vi "HFRR ADV v06 new software.vi"() -> ()   [LabVIEW 2025] (continued)
            frame 13 {
              n1278 = local write "CH-HEATER"(w1592) -> ()
            }
            frame 14 {
              n1279 = local write "CH-HUMIDITY WET"(w1593) -> ()
            }
            frame 15 {
              n1280 = local write "CH-HUMIDITY DRY"(w1594) -> ()
            }
            frame 16 {
            }
            frame 17 {
              n1281 = local write "AIR TEMP INTERCEPT:"(w1595) -> ()
            }
            frame 18 {
              n1282 = local write "TEMP INTERCEPT:"(w1596) -> ()
            }
            frame 19 {
              n1283 = local write "S.NO"(w1597) -> ()
            }
            frame 20 {
              n1284 = local write "Com Port 3"(w1598) -> ()
            }
            frame 21 {
            }
            frame 22 {
              n1285 = local write "C3 :"(w1599) -> ()
            }
            frame 23, Default {
            }
          }
        }
      }
    }
    n1286 = Select(t=u32 2500 ("milliseconds to wait"), s=w1553, f=u32 500 ("milliseconds to wait")) -> (s? t:f=w1551:u32)
    n1287 = Multiply(x=w1556, y=w1551) -> (x*y=w1558:dbl)
    n1288 = property on="Time slide" class="Slide (strict)"("Visible"=w1547) -> ()  [unwired: 2 in, 2 out]
    n1289 = call "Elapsed Time2"("Time Target (s)"=w1558, "Auto Reset"=TRUE) -> ("Time has Elapsed"=w1548:bool)  [unwired: 10 in, 7 out]
    n1290 = case shown="True" w1548 {
      frame False {
      }
      frame True {
        n1291 = stacked-sequence {
          frame #0 {
            # "DATA PROCESSING"
            # "115 mV/N"
            n1292 = local read "Sample Temperature"() -> (w1600:dbl)
            "TEMP 2" <- w1600
            "TEMP 3" <- w1600
            n1293 = local read "RH Numeric:"() -> (w1607:dbl)
            n1294 = local read "HUMIDITY:"() -> (w1608:dbl)
            n1295 = local read "FRICVALZ"() -> (w1619:dbl)
            n1296 = local read "Friction"() -> (w1603:dbl)
            n1297 = local write "TEMP"(w1600) -> ()
            n1298 = Multiply(x=w1607, y=w1608) -> (x*y=→"Humidity ( %RH )" →"Hum" →"Hum 2":dbl)
            n1299 = Subtract(x=w1603, y=w1619) -> (x-y=w1614:dbl)
            "FF 2" <- w1614
            "FF 4" <- w1614
            n1300 = local read "Ambient Temperature"() -> (→"AIR TEMP":dbl)
            n1301 = local read "TEMP"() -> (w1618:dbl)
            n1302 = local write "FF 3"(w1614) -> ()
            n1303 = Compound Arithmetic op=OR("FRICVALZ 4", "FRICVALZ 3", "FRICVALZ 2") -> (w1610:bool)
            n1304 = case shown="True" w1610 {
              tunnel: w1603 -> [_ w1625]
              frame False {
              }
              frame True {
                w1624 = FALSE ("FRICVALZ")
                n1305 = local write "FRICVALZ 3"(w1624) -> ()
                n1306 = local write "FRICVALZ 2"(w1624) -> ()
                n1307 = local write "FRICVALZ 4"(w1624) -> ()
                "FRICVALZ" <- w1625
              }
            }
            n1308 = Not A Number/Path/Refnum?(number/path/refnum=w1618) -> (NaN/Path/Refnum?=w1617:bool)
            n1309 = Not A Number/Path/Refnum?(number/path/refnum=w1614) -> (NaN/Path/Refnum?=w1616:bool)
            n1310 = Divide(x=w1614, y=1.96) -> (x/y=w1611:dbl)
            n1311 = Compound Arithmetic op=OR(w1617, w1616) -> (w1615:bool)
            n1312 = Not A Number/Path/Refnum?(number/path/refnum=w1611) -> (NaN/Path/Refnum?=w1612:bool)
            n1313 = case shown="True" w1615 {
              frame False {
              }
              frame True {
                n1314 = local write "TEMP"(0.0 ("TEMP")) -> ()
                n1315 = local write "FF 2"(0.0 ("FF 2")) -> ()
                n1316 = local write "reinit"(TRUE ("reinit")) -> ()
              }
            }
            n1317 = Select(t=0.0, s=w1612, f=w1611) -> (s? t:f=w1602:dbl)
            "COF 2" <- w1602
            n1318 = local write "COF 3"(w1602) -> ()
          }
        }
      }
    }
    n1319 = Wait (ms)(milliseconds to wait=u32 50) -> ()  [unwired: 1 out]
    n1320 = local read "Quit"() -> (w1540:bool)
    "Rate" <- 2500.0 ("No of Samples")
  }
  n1321 = while {
    tunnel: w57 -> [_]
    tunnel: [w1652] -> _
    tunnel: [w1628] -> w56
    i -> [w1652]
    stop <- w1628 stop-if-true
    # "C:\\LAB-IQ-NXT\\Scar View.exe"
    n1322 = local read "OK Button 16"() -> (w1641:bool)
    n1323 = local read "Main Tab"() -> (w1634:T2)
    n1324 = local read "service 3"() -> (w1635:bool)
    n1325 = local read "OPEN 6"() -> (w1637:bool)
    n1326 = local read "EDIT 2"() -> (w1639:bool)
    n1327 = flat-sequence {
      frame #0 {
        n1328 = local read "SAVE 2"() -> (w2254:bool)
        n1329 = stacked-sequence {
          frame #0 {
            n1330 = local read "EDIT"() -> (w2308:bool)
            n1331 = case shown="True" w2308 {
              tunnel: [u8 2 ("Disabled") u8 0 ("Disabled")] -> _
              frame False {
                w2310 = FALSE
                n1332 = local write "Password"("") -> ()
                n1333 = property on="SrvM CP" class="Bool (strict)"("Visible"=w2310) -> ()  [unwired: 2 in, 2 out]
                n1334 = property on="message" class="Str"("Visible"=w2310) -> ()  [unwired: 2 in, 2 out]
                n1335 = local write "x = y?"(w2310) -> ()
                n1336 = property on="Password" class="Str"("Visible"=w2310) -> ()  [unwired: 2 in, 2 out]
                n1337 = property on="ENTER THE NEW PASSWORD" class="Str"("Visible"=w2310) -> ()  [unwired: 2 in, 2 out]
                n1338 = property on="ENTER CURRENT PASSWORD" class="Str"("Visible"=w2310) -> ()  [unwired: 2 in, 2 out]
                n1339 = local write "SrvM CP"(w2310) -> ()
              }
              frame True {
                w2313 = TRUE
                n1340 = property on="SrvM CP" class="Bool (strict)"("Visible"=w2313) -> ()  [unwired: 2 in, 2 out]
                n1341 = property on="Password" class="Str"("Visible"=w2313) -> ()  [unwired: 2 in, 2 out]
              }
            }
            "dipl pwd" <- "@143$\n" ("dipl pwd")
          }
          frame #1 {
            # "Gain password"
            n1342 = String To Byte Array(string="ENTER CURRENT PASSWORD") -> (unsigned byte array=w2318:u8[])
            n1343 = Search 1D Array(1D array=w2318, element=u8 10) -> (index of element=w2321:i32)  [unwired: 1 in]
            n1344 = Index Array(array=w2318, index=w2321) -> (element=w2317:u8)
            n1345 = Equal?(x=w2317, y=10) -> (x = y?=w2315:bool)
            n1346 = case shown="True" w2315 {
              frame False {
                n1347 = property on="ENTER THE NEW PASSWORD" class="Str"("Visible"=FALSE) -> ()  [unwired: 2 in, 2 out]
              }
              frame True {
                # "password"
                # "change password logic"
                n1348 = local read "ENTER CURRENT PASSWORD"() -> (w2334:string)
                n1349 = local read "dipl pwd"() -> (w2328:string)
                n1350 = String To Byte Array(string=w2334) -> (unsigned byte array=w2336:u8[])
                n1351 = String To Byte Array(string=w2328) -> (unsigned byte array=w2329:u8[])
                n1352 = Array Size(array=w2336) -> (size(s)=w2333:i32)
                n1353 = Array Size(array=w2329) -> (size(s)=w2331:i32)
                n1354 = for {
                  N: w2333 -> [_]
                  tunnel: w2336 -> [w2360]
                  tunnel: [w2358] -> w2337 mode=indexing
                  tunnel: w2333 -> [w2352]
                  i -> [w2353]
                  n1355 = Decrement(x=w2352) -> (x-1=w2350:i32)
                  n1356 = Equal?(x=w2353, y=w2350) -> (x = y?=w2351:bool)
                  n1357 = Index Array(array=w2360, index=w2353) -> (element=w2354:u8)
                  n1358 = Number To Decimal String(number=w2354) -> (decimal integer string=w2359:string)  [unwired: 1 in]
                  n1359 = Select(t="", s=w2351, f="\r") -> (s? t:f=w2356:string)
                  n1360 = Concatenate Strings(w2359, w2356) -> (w2358:string)
                }
                n1361 = for {
                  N: w2331 -> [_]
                  tunnel: w2329 -> [w2348]
                  tunnel: [w2346] -> w2330 mode=indexing
                  tunnel: w2331 -> [w2343]
                  i -> [w2344]
                  n1362 = Decrement(x=w2343) -> (x-1=w2342:i32)
                  n1363 = Equal?(x=w2344, y=w2342) -> (x = y?=w2341:bool)
                  n1364 = Index Array(array=w2348, index=w2344) -> (element=w2347:u8)
                  n1365 = Number To Decimal String(number=w2347) -> (decimal integer string=w2345:string)  [unwired: 1 in]
                  n1366 = Select(t="", s=w2341, f="\r") -> (s? t:f=w2338:string)
                  n1367 = Concatenate Strings(w2345, w2338) -> (w2346:string)
                }
                n1368 = local read "string"() -> (w2335:string)
                n1369 = Concatenate Strings(w2330) -> (w2324:string)
                n1370 = Concatenate Strings(w2335) -> (w2332:string)
                n1371 = Concatenate Strings(w2337) -> (w2325:string)
                n1372 = Equal?(x=w2325, y=w2332) -> (x = y?=w2327:bool)
                n1373 = Equal?(x=w2325, y=w2324) -> (x = y?=w2323:bool)
                n1374 = Or(x=w2327, y=w2323) -> (x .or. y?=w2326:bool)
                n1375 = case shown="True" w2326 {
                  frame False {
                  }
                  frame True {
                    n1376 = property on="ENTER THE NEW PASSWORD" class="Str"("Visible"=TRUE) -> ()  [unwired: 2 in, 2 out]
                  }
                }
              }
            }
          }
          frame #2 {
            n1377 = String To Byte Array(string="ENTER THE NEW PASSWORD") -> (unsigned byte array=w2363:u8[])
            n1378 = Search 1D Array(1D array=w2363, element=u8 10) -> (index of element=w2367:i32)  [unwired: 1 in]
            n1379 = Index Array(array=w2363, index=w2367) -> (element=w2365:u8)
            n1380 = Equal?(x=w2365, y=10) -> (x = y?=w2362:bool)
            n1381 = case shown="False" w2362 {
              frame False {
              }
              frame True {
                n1382 = local write "EDIT"(FALSE) -> ()
                n1383 = local write "SrvM CP"(FALSE) -> ()
                n1384 = local read "ENTER THE NEW PASSWORD"() -> (w2370:string)
                n1385 = String To Byte Array(string=w2370) -> (unsigned byte array=w2375:u8[])
                n1386 = Array Size(array=w2375) -> (size(s)=w2372:i32)
                n1387 = for {
                  N: w2372 -> [_]
                  tunnel: w2375 -> [w2388]
                  tunnel: [w2385] -> w2377 mode=indexing
                  tunnel: w2372 -> [w2380]
                  i -> [w2378]
                  n1388 = Decrement(x=w2380) -> (x-1=w2381:i32)
                  n1389 = Equal?(x=w2378, y=w2381) -> (x = y?=w2382:bool)
                  n1390 = Index Array(array=w2388, index=w2378) -> (element=w2387:u8)
                  n1391 = Number To Decimal String(number=w2387) -> (decimal integer string=w2386:string)  [unwired: 1 in]
                  n1392 = Select(t="", s=w2382, f="\r") -> (s? t:f=w2379:string)
                  n1393 = Concatenate Strings(w2386, w2379) -> (w2385:string)
                }
                n1394 = local read "file path"() -> (w2369:path)
                n1395 = Concatenate Strings(w2377) -> (w2371:string)
                n1396 = Delete(path (use dialog)=w2369) -> (deleted path=w2373:path)  [unwired: 4 in, 2 out]
                n1397 = call <vilib>:"Write Characters To File.vi"("append to file? (new file:F)"=FALSE, "character string"=w2371, "file path (dialog if empty)"=w2373) -> ()  [unwired: 2 in, 1 out]
              }
            }
          }
          frame #3 {
            n1398 = case shown="True" "SrvM CP" {
              frame False {
                w2391 = ""
                n1399 = local write "ENTER CURRENT PASSWORD"(w2391) -> ()
                n1400 = local write "ENTER THE NEW PASSWORD"(w2391) -> ()
                n1401 = property on="ENTER CURRENT PASSWORD" class="Str"("Visible"=FALSE) -> ()  [unwired: 2 in, 2 out]
              }
              frame True {
                n1402 = property on="ENTER THE NEW PASSWORD" class="Str"() -> ("Visible"=w2392:bool)  [unwired: 2 in, 2 out]
                n1403 = Not(x=w2392) -> (.not. x?=w2393:bool)
                n1404 = property on="ENTER CURRENT PASSWORD" class="Str"("Visible"=w2393) -> ()  [unwired: 2 in, 2 out]
              }
            }
          }
          frame #4 {
            n1405 = String To Byte Array(string="Password") -> (unsigned byte array=w2400:u8[])
            n1406 = Search 1D Array(1D array=w2400, element=u8 10) -> (index of element=w2398:i32)  [unwired: 1 in]
            n1407 = Index Array(array=w2400, index=w2398) -> (element=w2399:u8)
            n1408 = Equal?(x=w2399, y=10) -> (x = y?=w2395:bool)
            n1409 = case shown="True" w2395 {
              frame False {
              }
              frame True {
                # "password"
                # "password"
                n1410 = local read "Password"() -> (w2413:string)
                n1411 = String To Byte Array(string=w2413) -> (unsigned byte array=w2416:u8[])
                n1412 = String To Byte Array(string="@143$\n") -> (unsigned byte array=w2402:u8[])
                n1413 = Array Size(array=w2416) -> (size(s)=w2411:i32)
                n1414 = Array Size(array=w2402) -> (size(s)=w2407:i32)
                n1415 = for {
                  N: w2411 -> [_]
                  tunnel: w2416 -> [w2450]
                  tunnel: [w2448] -> w2417 mode=indexing
                  tunnel: w2411 -> [w2445]
                  i -> [w2446]
                  n1416 = Decrement(x=w2445) -> (x-1=w2444:i32)
                  n1417 = Index Array(array=w2450, index=w2446) -> (element=w2449:u8)
                  n1418 = Equal?(x=w2446, y=w2444) -> (x = y?=w2443:bool)
                  n1419 = Number To Decimal String(number=w2449) -> (decimal integer string=w2447:string)  [unwired: 1 in]
                  n1420 = Select(t="", s=w2443, f="\r") -> (s? t:f=w2440:string)
                  n1421 = Concatenate Strings(w2447, w2440) -> (w2448:string)
                }
                n1422 = for {
                  N: w2407 -> [_]
                  tunnel: w2402 -> [w2461]
                  tunnel: [w2459] -> w2405 mode=indexing
                  tunnel: w2407 -> [w2456]
                  i -> [w2457]
                  n1423 = Decrement(x=w2456) -> (x-1=w2455:i32)
                  n1424 = Index Array(array=w2461, index=w2457) -> (element=w2460:u8)
                  n1425 = Equal?(x=w2457, y=w2455) -> (x = y?=w2454:bool)
                  n1426 = Number To Decimal String(number=w2460) -> (decimal integer string=w2458:string)  [unwired: 1 in]
                  n1427 = Select(t="", s=w2454, f="\r") -> (s? t:f=w2451:string)
                  n1428 = Concatenate Strings(w2458, w2451) -> (w2459:string)
                }
                n1429 = local read "file path"() -> (w2401:path)
                n1430 = call <vilib>:"Read Characters From File.vi"("file path (dialog if empty)"=w2401) -> ("character string"=w2415:string)  [unwired: 5 in, 3 out]
                "string" <- w2415
                n1431 = flat-sequence {
                  tunnel: [w2418] -> w2412
                  frame #0 {
                    w2418 = ""
                    n1432 = local write "Password"(w2418) -> ()
                  }
                }
                n1433 = Concatenate Strings(w2405) -> (w2406:string)
                n1434 = Concatenate Strings(w2415) -> (w2414:string)
                n1435 = Concatenate Strings(w2417) -> (w2409:string)
                n1436 = Equal?(x=w2409, y=w2414) -> (x = y?=w2404:bool)
                n1437 = Equal?(x=w2409, y=w2406) -> (x = y?=w2410:bool)
                n1438 = Or(x=w2404, y=w2410) -> (x .or. y?=w2403:bool)
                "x = y?" <- w2403
                n1439 = case shown="True" w2403 {
                  selector: w2403 -> [w2420 _]
                  tunnel: w2412 -> [_ _]
                  frame False {
                    n1440 = And(x=w2420, y=TRUE ("Visible")) -> (x .and. y?=w2421:bool)
                    n1441 = property on="message" class="Str"("Visible"=w2421) -> ()  [unwired: 2 in, 2 out]
                  }
                  frame True {
                    n1442 = control-ref of="This VI"() -> (w2432:refnum<vi>)
                    n1443 = property class="VI"(reference=w2432) -> (reference out=w2423:refnum<vi>, error out=w2427:errorcluster, "Panel"=w2431:refnum<vi>)  [unwired: 1 in]
                    n1444 = property on="message" class="Str"("Visible"=FALSE) -> ()  [unwired: 2 in, 2 out]
                    n1445 = property class="Pnl"(reference=w2431, error in=w2427) -> (reference out=w2425:refnum<vi>, error out=w2428:errorcluster, "Panes[]"=w2430:refnum<vi>[])
                    n1446 = for {
                      tunnel: w2430 -> [w2439] mode=indexing
                      tunnel: T16."Always On" ("Horizontal Scrollbar Visibility") -> [w2438]
                      tunnel: w2428 -> [w2435]
                      tunnel: [w2434] -> w2426
                      n1447 = property class="Pane"(reference=w2439, error in=w2435, "HorizScrollbarVisibility"=w2438) -> (reference out=w2436:refnum<vi>, error out=w2437:errorcluster)
                      n1448 = Close Reference(reference=w2436, error in (no error)=w2437) -> (error out=w2434:errorcluster)
                    }
                    n1449 = Close Reference(reference=w2425, error in (no error)=w2426) -> (error out=w2424:errorcluster)
                    n1450 = Close Reference(reference=w2423, error in (no error)=w2424) -> (error out=→"error out 6":errorcluster)
                  }
                }
              }
            }
          }
        }
        n1451 = local read "x = y?"() -> (w2260:bool)
        n1452 = local read "HUMIDITY: 2"() -> (w2262:dbl)
        n1453 = local read "HUMIDITY:"() -> (w2261:dbl)
        n1454 = property on="Port 2 Error" class="Clust (strict)"("Visible"="EDIT") -> ()  [unwired: 2 in, 2 out]
        n1455 = property on="Port 1 Error" class="Clust (strict)"("Visible"="EDIT") -> ()  [unwired: 2 in, 2 out]
        n1456 = case shown="True" "SrvM CP 2" {
          frame False {
          }
          frame True {
            n1457 = local write "SrvM CP 2"(FALSE ("SrvM CP 2")) -> ()
            n1458 = local read "HUMIDITY: 2"() -> (w2301:dbl)
            n1459 = local read "TEMP INTERCEPT: 2"() -> (w2300:dbl)
            n1460 = local read "DISPLACEMENT : 4"() -> (w2304:dbl)
            n1461 = local read "TEMPERATURE : 2"() -> (w2303:dbl)
            n1462 = local read "STROKE GAIN : 2"() -> (w2305:dbl)
            n1463 = local read "FRIC. FORCE : 2"() -> (w2306:dbl)
            n1464 = local read "AIR TEMP INTERCEPT: 2"() -> (w2299:dbl)
            n1465 = local read "AIR TEMPERATURE : 2"() -> (w2302:dbl)
            n1466 = local write "HUMIDITY:"(w2301) -> ()
            n1467 = local write "AIR TEMP INTERCEPT:"(w2300) -> ()
            n1468 = local write "TEMPERATURE :"(w2303) -> ()
            n1469 = local write "FRIC. FORCE :"(w2306) -> ()
            n1470 = local write "STROKE GAIN :"(w2305) -> ()
            n1471 = local write "DISPLACEMENT :"(w2304) -> ()
            n1472 = local write "AIR TEMPERATURE :"(w2302) -> ()
            n1473 = local write "TEMP INTERCEPT:"(w2299) -> ()
          }
        }
        n1474 = Or(x="SAVE", y=w2254) -> (x .or. y?=w2255:bool)
        n1475 = And(x="EDIT", y=w2260) -> (x .and. y?=w2258:bool)
        n1476 = local read "DISPLACEMENT : 4"() -> (w2271:dbl)
        n1477 = local read "TEMPERATURE : 2"() -> (w2269:dbl)
        n1478 = local read "STROKE GAIN : 2"() -> (w2275:dbl)
        n1479 = local read "DISPLACEMENT :"() -> (w2270:dbl)
        n1480 = local read "FRIC. FORCE : 2"() -> (w2278:dbl)
        n1481 = local read "TEMPERATURE :"() -> (w2267:dbl)
        n1482 = local read "STROKE GAIN :"() -> (w2274:dbl)
        n1483 = local read "FRIC. FORCE :"() -> (w2277:dbl)
        n1484 = case shown="True" w2258 {
          tunnel: [u8 2 ("Disabled") u8 0 ("Disabled")] -> w2257
          tunnel: [w2622 TRUE ("Visible")] -> w2256
          frame False {
            w2622 = FALSE ("Visible")
            n1485 = local write "EDIT 2"(w2622) -> ()
          }
          frame True {
          }
        }
        n1486 = case shown="True" w2255 {
          frame False {
          }
          frame True {
            n1487 = stacked-sequence {
              seq-local: [w2470 _ _] -> [_ w2617 _]
              frame #0 {
                (unwired) i16 5 ("precision (6)")
                # "[CH1]    - FF\n[CH2]   - TEMPERATURE\n[CH3]    - Humidity\n[CH4]    - AIR TEMP\n[CH5]\\- Visa Uno\n[CH6] \\- Visa Due\n[CH7]  \\- file path\n[CH8]   - Displacement Gain\n[CHA]   - Stroke Gain\n[CHB]   - Stroke PID Gain\n[CHC]   -Language Selection\n[CHD]   -Power +\n[CHE]   -Power_\n[CHF]   -Heater\n[CHG]   -Humidity Wet\n[CHH]   -Humidity Dry\n[CHI]   -Integral Time"
                n1488 = local read "Language Selection"() -> (w2518:enum16{"English", "Russian"})
                n1489 = local read "CH-HUMIDITY WET"() -> (w2476:u16)
                n1490 = local read "CH-HUMIDITY DRY"() -> (w2473:u16)
                n1491 = local read "STROKE GAIN :"() -> (w2462:dbl)
                n1492 = local read "CH-POWER +"() -> (w2485:u16)
                n1493 = local read "CH-POWER -"() -> (w2482:u16)
                n1494 = local read "CH-HEATER"() -> (w2479:u16)
                n1495 = local read "AIR TEMPERATURE :"() -> (w2465:dbl)
                n1496 = local read "DISPLACEMENT :"() -> (w2463:dbl)
                n1497 = local read "TEMPERATURE :"() -> (w2466:dbl)
                n1498 = local read "FRIC. FORCE :"() -> (w2467:dbl)
                n1499 = local read "HUMIDITY:"() -> (w2464:dbl)
                n1500 = Path To String(path="File Path") -> (string=w2534:string)
                n1501 = Number To Fractional String(number=w2462, width (-)=i16 10 ("precision (6)"), precision (6)=i16 5) -> (F-format string=w2525:string)  [unwired: 1 in]
                n1502 = Number To Fractional String(number=w2518, width (-)=i16 10 ("precision (6)"), precision (6)=i16 5) -> (F-format string=w2514:string)  [unwired: 1 in]
                n1503 = Number To Fractional String(number=w2485, width (-)=i16 10 ("precision (6)"), precision (6)=i16 5) -> (F-format string=w2508:string)  [unwired: 1 in]
                n1504 = Number To Fractional String(number=w2482, width (-)=i16 10 ("precision (6)"), precision (6)=i16 5) -> (F-format string=w2505:string)  [unwired: 1 in]
                n1505 = Number To Fractional String(number=w2479, width (-)=i16 10 ("precision (6)"), precision (6)=i16 5) -> (F-format string=w2500:string)  [unwired: 1 in]
                n1506 = Number To Fractional String(number=w2476, width (-)=i16 10 ("precision (6)"), precision (6)=i16 5) -> (F-format string=w2497:string)  [unwired: 1 in]
                n1507 = Number To Fractional String(number=w2473, width (-)=i16 10 ("precision (6)"), precision (6)=i16 5) -> (F-format string=w2492:string)  [unwired: 1 in]
                n1508 = local read "Com Port 1"() -> (w2469:refnum<visa-resource-name>)
                n1509 = local read "Com Port 2"() -> (w2468:refnum<visa-resource-name>)
                n1510 = Concatenate Strings(w2534, "\\" ("string")) -> (w2533:string)
                n1511 = Number To Fractional String(number=w2467, width (-)=i16 10 ("precision (6)"), precision (6)=i16 5) -> (F-format string=w2566:string)  [unwired: 1 in]
                n1512 = Number To Fractional String(number=w2466, width (-)=i16 10 ("precision (6)"), precision (6)=i16 5) -> (F-format string=w2565:string)  [unwired: 1 in]
                n1513 = Number To Fractional String(number=w2464, width (-)=i16 10 ("precision (6)"), precision (6)=i16 5) -> (F-format string=w2559:string)  [unwired: 1 in]
                n1514 = Number To Fractional String(number=w2465, width (-)=i16 10 ("precision (6)"), precision (6)=i16 5) -> (F-format string=w2553:string)  [unwired: 1 in]
                n1515 = Number To Fractional String(number=w2463, width (-)=i16 10 ("precision (6)"), precision (6)=i16 5) -> (F-format string=w2526:string)  [unwired: 1 in]
                n1516 = Concatenate Strings("[CHA]" ("string"), w2525, "- Stroke Gain" ("string"), "\r") -> (w2519:string)
                n1517 = Concatenate Strings("[CHC]" ("string"), w2514, "-Language Selection" ("string"), "\r") -> (w2511:string)
                n1518 = Concatenate Strings("[CHD]" ("string"), w2508, "-Power +" ("string"), "\r") -> (w2490:string)
                n1519 = Concatenate Strings("[CHG]" ("string"), w2497, "-Humidity Wet" ("string"), "\r") -> (w2487:string)
                n1520 = Concatenate Strings("[CHH]" ("string"), w2492, "-Humidity Dry" ("string"), "\r") -> (w2486:string)
                n1521 = Concatenate Strings("[CH1]" ("string"), w2566, " - FF" ("string"), "\r") -> (w2564:string)
                n1522 = Concatenate Strings("[CH2]" ("string"), w2565, " - TEMPERATURE" ("string"), "\r") -> (w2563:string)
                n1523 = Concatenate Strings("[CH3]" ("string"), w2559, " - Humidity" ("string"), "\r") -> (w2556:string)
                n1524 = Concatenate Strings("[CH4]" ("string"), w2553, " - AIR TEMP" ("string"), "\r") -> (w2549:string)
                n1525 = Concatenate Strings("[CH5]" ("string"), w2469, "- Visa Uno" ("string"), "\r") -> (w2542:string)
                n1526 = Concatenate Strings("[CH6]" ("string"), w2468, "- Visa Due" ("string"), "\r") -> (w2537:string)
                n1527 = Concatenate Strings("[CH7]" ("string"), w2533, "- file path" ("string"), "\r") -> (w2536:string)
                n1528 = Concatenate Strings("[CH8]" ("string"), w2526, "- Displacement Gain" ("string"), "\r") -> (w2529:string)
                n1529 = Concatenate Strings("[CHE]" ("string"), w2505, "-Power_" ("string"), "\r") -> (w2489:string)
                n1530 = Concatenate Strings("[CHF]" ("string"), w2500, "-Heater" ("string"), "\r") -> (w2488:string)
                n1531 = Concatenate Strings(w2564, w2563, w2556, w2549, w2542, w2537, w2536, w2529, w2519, w2511, w2490, w2489, w2488, w2487, w2486) -> (w2470:string)
                "gain" <- w2470
              }
              frame #1 {
                n1532 = local read "Camera Port :"() -> (w2578:string)
                n1533 = local read "C3 :"() -> (w2586:refnum<visa-resource-name>)
                n1534 = local read "TEMP INTERCEPT:"() -> (w2587:dbl)
                n1535 = local read "AIR TEMP INTERCEPT:"() -> (w2588:dbl)
                n1536 = Concatenate Strings("[CH8]" ("string"), w2578, "- Visa Camera" ("string"), "\r") -> (w2577:string)
                n1537 = Concatenate Strings("[CH7]" ("string"), w2586, "- Visa Humidity" ("string"), "\r") -> (w2582:string)
                n1538 = Number To Fractional String(number=w2587, width (-)=i16 10 ("precision (6)"), precision (6)=i16 5) -> (F-format string=w2605:string)  [unwired: 1 in]
                n1539 = local read "Com Port 3"() -> (w2589:refnum<visa-resource-name>)
                n1540 = Number To Fractional String(number=w2588, width (-)=i16 10 ("precision (6)"), precision (6)=i16 5) -> (F-format string=w2612:string)  [unwired: 1 in]
                n1541 = Concatenate Strings("[CHK]" ("string"), w2605, "-TEMP INTERCEPT" ("string"), "\r") -> (w2601:string)
                n1542 = Concatenate Strings("[SNO]" ("string"), "S.NO", "-" ("string"), "\r") -> (w2597:string)
                n1543 = Concatenate Strings("[CHJ]" ("string"), w2612, "-AIR TEMP INTERCEPT" ("string"), "\r") -> (w2602:string)
                n1544 = Concatenate Strings("[CHL]" ("string"), w2589, "- Visa humid" ("string"), "\r") -> (w2592:string)
                n1545 = String To Path(string="C:\\LAB-IQ\\calibrate WO 2465.dcf") -> (path=w2590:path)
                n1546 = Concatenate Strings(w2617, w2602, w2601, w2597, w2592, w2582, w2577) -> (w2616:string)
                n1547 = call <vilib>:"Write Characters To File.vi"("append to file? (new file:F)"=FALSE, "character string"=w2616, "file path (dialog if empty)"=w2590) -> ()  [unwired: 2 in, 1 out]
              }
              frame #2 {
                n1548 = local write "Lan flag"(0.0 ("Lan flag")) -> ()
                n1549 = local write "conststatus"(0.0 ("rpm value : 2")) -> ()
                n1550 = local write "SAVE"(FALSE ("OK Button 14")) -> ()
                n1551 = local write "SAVE 2"(FALSE ("SAVE 2")) -> ()
              }
            }
          }
        }
        n1552 = Subtract(x=w2262, y=w2261) -> (x-y=w2263:dbl)
        n1553 = local read "AIR TEMPERATURE : 2"() -> (w2266:dbl)
        n1554 = local read "AIR TEMPERATURE :"() -> (w2265:dbl)
        n1555 = Divide(x=w2263, y=w2261) -> (x/y=w2285:dbl)
        n1556 = Subtract(x=w2278, y=w2277) -> (x-y=w2276:dbl)
        n1557 = Subtract(x=w2269, y=w2267) -> (x-y=w2268:dbl)
        n1558 = Subtract(x=w2275, y=w2274) -> (x-y=w2273:dbl)
        n1559 = Subtract(x=w2271, y=w2270) -> (x-y=w2272:dbl)
        n1560 = Subtract(x=w2266, y=w2265) -> (x-y=w2264:dbl)
        n1561 = Divide(x=w2276, y=w2277) -> (x/y=w2296:dbl)
        n1562 = Divide(x=w2268, y=w2267) -> (x/y=w2289:dbl)
        n1563 = Divide(x=w2273, y=w2274) -> (x/y=w2293:dbl)
        n1564 = Divide(x=w2272, y=w2270) -> (x/y=w2292:dbl)
        n1565 = Multiply(x=w2285, y=100.0) -> (x*y=→"HUMIDITY  Calibration Error":dbl)
        n1566 = Divide(x=w2264, y=w2265) -> (x/y=w2288:dbl)
        n1567 = Multiply(x=w2296, y=100.0) -> (x*y=→"FRIC. FORCE Calibration Error":dbl)
        n1568 = Multiply(x=w2289, y=100.0) -> (x*y=→"TEMPERATURE  Calibration Error":dbl)
        n1569 = Multiply(x=w2293, y=100.0) -> (x*y=→"STROKE Calibration Error":dbl)
        n1570 = Multiply(x=w2292, y=100.0) -> (x*y=→"DISPLACEMENT  Calibration Error":dbl)
        n1571 = property on="EDIT 2" class="Bool (strict)"("Visible"=w2256) -> ()  [unwired: 2 in, 2 out]
        n1572 = property on="SAVE" class="Bool (strict)"("Visible"=w2256) -> ()  [unwired: 2 in, 2 out]
        n1573 = property on="SrvM CP" class="Bool (strict)"("Disabled"=w2257) -> ()  [unwired: 2 in, 2 out]
        n1574 = property on="visa due" class="CmbBox"("Disabled"=w2257) -> ()  [unwired: 2 in, 2 out]
        n1575 = property on="File Path" class="Path"("Disabled"=w2257) -> ()  [unwired: 2 in, 2 out]
        n1576 = Multiply(x=w2288, y=100.0) -> (x*y=→"AIR TEMPERATURE  Calibration Error":dbl)
        n1577 = property on="Language Selection" class="Enum (strict)"("Visible"=w2256) -> ()  [unwired: 2 in, 2 out]
        n1578 = property on="Tab Control 7" class="TabCtl (strict)"("Disabled"=w2257) -> ()  [unwired: 2 in, 2 out]
        n1579 = property on="AIR TEMP INTERCEPT:" class="DigNum (strict)"("Disabled"=w2257) -> ()  [unwired: 2 in, 2 out]
        n1580 = property on="CH-POWER -" class="DigNum (strict)"("Disabled"=w2257) -> ()  [unwired: 2 in, 2 out]
        n1581 = property on="CH-POWER +" class="DigNum (strict)"("Disabled"=w2257) -> ()  [unwired: 2 in, 2 out]
        n1582 = property on="AIR TEMPERATURE :" class="DigNum (strict)"("Disabled"=w2257) -> ()  [unwired: 2 in, 2 out]
        n1583 = property on="STROKE GAIN :" class="DigNum (strict)"("Disabled"=w2257) -> ()  [unwired: 2 in, 2 out]
        n1584 = property on="SPEED OUT:" class="DigNum (strict)"("Disabled"=w2257) -> ()  [unwired: 2 in, 2 out]
        n1585 = property on="CH-HUMIDITY DRY" class="DigNum (strict)"("Disabled"=w2257) -> ()  [unwired: 2 in, 2 out]
        n1586 = property on="HUMIDITY:" class="DigNum (strict)"("Disabled"=w2257) -> ()  [unwired: 2 in, 2 out]
        n1587 = property on="CH-HUMIDITY WET" class="DigNum (strict)"("Disabled"=w2257) -> ()  [unwired: 2 in, 2 out]
        n1588 = property on="TEMPERATURE :" class="DigNum (strict)"("Disabled"=w2257) -> ()  [unwired: 2 in, 2 out]
        n1589 = property on="DISPLACEMENT :" class="DigNum (strict)"("Disabled"=w2257) -> ()  [unwired: 2 in, 2 out]
        n1590 = property on="CH-HEATER" class="DigNum (strict)"("Disabled"=w2257) -> ()  [unwired: 2 in, 2 out]
        n1591 = property on="TEMP INTERCEPT:" class="DigNum (strict)"("Disabled"=w2257) -> ()  [unwired: 2 in, 2 out]
        n1592 = property on="FRIC. FORCE :" class="DigNum (strict)"("Disabled"=w2257) -> ()  [unwired: 2 in, 2 out]
      }
    }
    n1593 = local read "RUN"() -> (w1651:bool)
    n1594 = local read "RUN"() -> (w1649:bool)
    n1595 = disable-structure shown="Disabled" {
      disable-tunnel: [w1666 _] -> w1632
      disable-tunnel: [w1665 _] -> w1630
      frame Disabled {
        n1596 = local read "Temperature before test"() -> (w1659:dbl)
        n1597 = local read "Temperature after test"() -> (w1672:dbl)
        n1598 = case shown="True" "Save Results" {
          frame False {
          }
          frame True {
            w1688 = "\r"
            n1599 = local write "Save Results"(FALSE ("OK Button 5")) -> ()
            n1600 = local read "Temperature before test"() -> (w1726:dbl)
            n1601 = local read "Temperature after test"() -> (w1728:dbl)
            n1602 = local read "Humidity before test"() -> (w1725:dbl)
            n1603 = local read "Humidity after test"() -> (w1727:dbl)
            n1604 = local read "WS1.4"() -> (w1732:dbl)
            n1605 = local read "AVP"() -> (w1730:dbl)
            n1606 = Number To Fractional String(number=w1732, width (-)=i16 6, precision (6)=i16 1) -> (F-format string=w1692:string)  [unwired: 1 in]
            n1607 = local read "MWSD"() -> (w1729:dbl)
            n1608 = local read "String"() -> (w1721:string)
            n1609 = local read "FILE"() -> (w1724:string)
            n1610 = local read "HCF"() -> (w1731:dbl)
            n1611 = Number To Fractional String(number=w1725, width (-)=i16 6, precision (6)=i16 1) -> (F-format string=w1717:string)  [unwired: 1 in]
            n1612 = Number To Fractional String(number=w1726, width (-)=i16 6, precision (6)=i16 1) -> (F-format string=w1714:string)  [unwired: 1 in]
            n1613 = Number To Fractional String(number=w1727, width (-)=i16 6, precision (6)=i16 1) -> (F-format string=w1710:string)  [unwired: 1 in]
            n1614 = Number To Fractional String(number=w1728, width (-)=i16 6, precision (6)=i16 1) -> (F-format string=w1706:string)  [unwired: 1 in]
            n1615 = Number To Fractional String(number=w1730, width (-)=i16 6, precision (6)=i16 3) -> (F-format string=w1699:string)  [unwired: 1 in]
            n1616 = Concatenate Strings(w1721, w1724) -> (w1743:string)
            n1617 = Number To Fractional String(number=w1729, width (-)=i16 6, precision (6)=i16 1) -> (F-format string=w1703:string)  [unwired: 1 in]
            n1618 = Number To Fractional String(number=w1731, width (-)=i16 6, precision (6)=i16 2) -> (F-format string=w1697:string)  [unwired: 1 in]
            n1619 = Concatenate Strings("(" ("string"), w1692, ")Microns" ("string")) -> (w1691:string)
            n1620 = local read "REMARKS"() -> (w1723:string)
            "REMARKS 2" <- w1723
            n1621 = Concatenate Strings("(" ("string"), w1717, " ) % RH," ("string")) -> (w1718:string)
            n1622 = Concatenate Strings(w1697, ")" ("string")) -> (w1695:string)
            n1623 = Concatenate Strings("(" ("string"), w1714, ")  Deg C ," ("string")) -> (w1713:string)
            n1624 = Concatenate Strings("(" ("string"), w1710, " ) % RH," ("string")) -> (w1709:string)
            n1625 = Concatenate Strings("(" ("string"), w1706, ")  Deg C ," ("string")) -> (w1705:string)
            n1626 = Concatenate Strings("(" ("string"), w1703, ")  Microns," ("string")) -> (w1702:string)
            n1627 = Concatenate Strings("(" ("string"), w1699, ")  kPa," ("string")) -> (w1689:string)
            n1628 = Concatenate Strings(w1743, ".dwm" ("Substring")) -> (w1741:string)
            n1629 = String To Path(string=w1741) -> (path=w1740:path)
            n1630 = Concatenate Strings(w1723, w1688, " Humidity before test= " ("Substring"), w1718, w1688, " Temperature before test = " ("Substring"), w1713, w1688, " Humidity after test= " ("Substring"), w1709, w1688, "Temperature after test = " ("Substring"), w1705, w1688, "MSD = " ("Substring"), w1702, w1688, "  AVP = " ("Substring"), w1689, w1688, "  HCF                     =( " ("Substring"), w1695, w1688, " WS1.4                  = " ("Substring"), w1691, w1688) -> (w1687:string)
            "data" <- w1687
            n1631 = call <vilib>:"Write Characters To File.vi"("append to file? (new file:F)"=FALSE, "character string"=w1687, "file path (dialog if empty)"=w1740) -> ()  [unwired: 2 in, 1 out]
            n1632 = Match Pattern(string=w1687, regular expression="!") -> (after substring=→"export":string)  [unwired: 1 in, 3 out]
          }
        }
        n1633 = Add(x=231.864, y=w1659) -> (x+y=w1656:dbl)
        n1634 = Add(x=231.864, y=w1672) -> (x+y=w1669:dbl)
        n1635 = Divide(x=1705.984, y=w1656) -> (x/y=w1657:dbl)
        n1636 = Divide(x=1705.984, y=w1669) -> (x/y=w1670:dbl)
        n1637 = local read "Humidity before test"() -> (w1661:dbl)
        n1638 = local read "Humidity after test"() -> (w1674:dbl)
        n1639 = Subtract(x=8.017352 ("y"), y=w1657) -> (x-y=w1683:dbl)
        n1640 = Subtract(x=8.017352 ("y"), y=w1670) -> (x-y=w1677:dbl)
        n1641 = expression code="10**y"(w1683) -> (w1663:dbl)
        n1642 = expression code="10**y"(w1677) -> (w1676:dbl)
        n1643 = Multiply(x=w1661, y=w1663) -> (x*y=w1662:dbl)
        n1644 = Multiply(x=w1674, y=w1676) -> (x*y=w1675:dbl)
        n1645 = Divide(x=w1662, y=750.0) -> (x/y=w1678:dbl)
        n1646 = Divide(x=w1675, y=750.0) -> (x/y=w1679:dbl)
        n1647 = Add(x=w1678, y=w1679) -> (x+y=w1680:dbl)
        n1648 = Divide(x=w1680, y=2.0) -> (x/y=w1682:dbl)
        n1649 = local write "AVP"(w1682) -> ()
        n1650 = Subtract(x=1.4, y=w1682) -> (x-y=w1665:dbl)
        n1651 = local read "HCF"() -> (w1666:dbl)
      }
      frame Enabled {
      }
    }
    n1652 = case shown="True" "EDIT 3" {
      frame False {
      }
      frame True {
        n1653 = local write "EDIT 3"(FALSE ("EDIT 3")) -> ()
        n1654 = local write "Main Tab"(T2."About" ("Main Tab")) -> ()
      }
    }
    n1655 = case shown="False" w1651 {
      frame False {
        n1656 = local read "stopT"() -> (w2629:bool)
        n1657 = case shown="True" w2629 {
          frame False {
          }
          frame True {
            n1658 = local write "stopT"(FALSE) -> ()
          }
        }
      }
      frame True {
        "stopT" <- TRUE
      }
    }
    n1659 = case shown="False" w1649 {
      frame False {
      }
      frame True {
      }
    }
    n1660 = case shown="True" w1639 {
      frame False {
        n1661 = property on="Password 2" class="Str"("Visible"=FALSE) -> ()  [unwired: 2 in, 2 out]
        n1662 = local write "Password 2"("" ("Password")) -> ()
      }
      frame True {
        n1663 = property on="Password 2" class="Str"("Visible"=TRUE) -> ()  [unwired: 2 in, 2 out]
        n1664 = Equal?(x="Password 2", y="HFRR1234") -> (x = y?=w1771:bool)
        n1665 = case shown="True" w1771 {
          tunnel: "Password 2" -> [w1774 _]
          frame False {
            n1666 = String Length(string=w1774) -> (length=w1775:i32)
            n1667 = Greater Than 0?(x=w1775) -> (x > 0?=w1773:bool)
            n1668 = case shown="False" w1773 {
              frame False {
                n1669 = property on="Password 2" class="Str"("Caption.Text"="Password (Advance Setting)") -> ()  [unwired: 2 in, 2 out]
              }
              frame True {
                n1670 = property on="Password 2" class="Str"("Caption.Text"="Incorrect Password!") -> ()  [unwired: 2 in, 2 out]
              }
            }
          }
          frame True {
            n1671 = local write "EDIT 2"(FALSE ("EDIT 2")) -> ()
            n1672 = local write "Password 2"("" ("Password")) -> ()
            n1673 = local write "Main Tab"(T2."Advance" ("Main Tab")) -> ()
            n1674 = local write "Main Dashboard Buttons"(T1."Advance" ("Main Dashboard Buttons")) -> ()
          }
        }
      }
    }
    n1675 = case shown="True" "Prog Uno" {
      frame False {
      }
      frame True {
        n1676 = stacked-sequence {
          frame #0 {
            n1677 = Delete(path (use dialog)=path "C:/LAB-IQ-NXT/UNOCOMPILE.bat" ("working directory")) -> ()  [unwired: 4 in, 3 out]
          }
          frame #1 {
            n1678 = local read "Com Port 1"() -> (w2236:refnum<visa-resource-name>)
            n1679 = Concatenate Strings("cmd.exe /c \"mode " ("command line"), w2236, ":1200,n,8,1\"\n" ("command line")) -> (w2241:string)
            n1680 = Concatenate Strings(w2241, "CD\\\nCD WinDucom\navrdude -C avrdude.conf -v -patmega328p -carduino -P" ("command line"), w2236, " -b115200 -D -Uflash:w:UNO_V20.hex:i\n" ("command line"), "\r") -> (w2243:string)
            "STR" <- w2243
            n1681 = call <vilib>:"Write Characters To File.vi"("append to file? (new file:F)"=FALSE, "character string"=w2243, "file path (dialog if empty)"=path "C:/LAB-IQ/UNOCOMPILE.bat" ("working directory")) -> ()  [unwired: 2 in, 1 out]
          }
          frame #2 {
            n1682 = disable-structure shown="Disabled" {
              frame Disabled {
                w2247 = "cmd.exe  /c \"C:\\LAB-IQ-NXT\\UNOCOMPILE.bat\"" ("string")
                n1683 = local write "Prog Uno"(FALSE ("run minimized? (F)")) -> ()
                n1684 = call <vilib>:"System Exec.vi"("expected output size  (4096)"=u32 65535, "run minimized? (F)"=FALSE, "wait until completion? (T)"=TRUE ("run minimized? (F)"), "working directory"=path "C:/LAB-IQ-NXT", "standard input"=w2247, "command line"=w2247) -> ("error out"=w2246:errorcluster, "standard output"=→"String 42":string)  [unwired: 2 in, 2 out]
                "error out 3" <- w2246
                n1685 = flat-sequence {
                  tunnel: w2246 -> [_]
                  frame #0 {
                  }
                }
              }
              frame Enabled {
              }
            }
          }
        }
      }
    }
    n1686 = case shown="\"ISO 12156\"" "TEST STANDARD" {
      tunnel: [2.0 ("Set Temp") 0.0 ("Set Temp") 2.0 ("Set Temp") 0.0 ("Set Temp")] -> w1640
      frame "ASTM D6079", Default {
        w2193 = 50.0 ("Hz")
        w2194 = 53.0 ("Set Rh")
        w2196 = 1.0 ("Set Strk")
        w2195 = 60.0 ("Set Temp")
        # "astm hide"
        n1687 = local write "NORMAL LOAD"(200.0 ("NORMAL LOAD")) -> ()
        n1688 = local write "Set Strk"(w2196) -> ()
        n1689 = local write "Set Hz"(w2193) -> ()
        n1690 = local write "Set Temp"(w2195) -> ()
        n1691 = local write "Set Rh"(w2194) -> ()
        n1692 = local write "test time"(75.0 ("test time")) -> ()
        n1693 = local write "Set Stroke:"(w2196) -> ()
        n1694 = local write "Set Humidity:"(w2194) -> ()
        n1695 = local write "Set Frequency:"(w2193) -> ()
        n1696 = local write "Set Temperature:"(w2195) -> ()
        "Test Standard" <- "ASTM D6079" ("Test Standard 2")
      }
      frame "ISO 12156" {
        n1697 = local write "Set Strk"(1.0 ("Set Strk")) -> ()
        n1698 = local write "NORMAL LOAD"(200.0 ("NORMAL LOAD")) -> ()
        n1699 = local write "Set Temp"(60.0 ("Set Temp")) -> ()
        n1700 = local write "test time"(75.0 ("test time")) -> ()
        n1701 = local write "Set Hz"(50.0 ("Hz")) -> ()
        n1702 = local write "Set Rh"(53.0 ("Set Rh")) -> ()
      }
      frame "CEC F-096-A-06" {
        n1703 = local write "Set Strk"(1.0 ("Set Strk")) -> ()
        n1704 = local write "NORMAL LOAD"(200.0 ("NORMAL LOAD")) -> ()
        n1705 = local write "Set Temp"(60.0 ("Set Temp")) -> ()
        n1706 = local write "test time"(75.0 ("test time")) -> ()
        n1707 = local write "Set Hz"(50.0 ("Hz")) -> ()
        n1708 = local write "Set Rh"(53.0 ("Set Rh")) -> ()
      }
      frame "Custom" {
      }
    }
    n1709 = case shown="True" "Prog Due" {
      frame False {
      }
      frame True {
        n1710 = stacked-sequence {
          frame #0 {
            n1711 = Delete(path (use dialog)=path "C:/LAB-IQ/DUECOMPILE.bat" ("working directory")) -> ()  [unwired: 4 in, 3 out]
          }
          frame #1 {
            n1712 = disable-structure shown="Disabled" {
              frame Disabled {
                n1713 = local read "visa due"() -> (w2218:string)
                n1714 = Concatenate Strings("cmd.exe /c \"mode " ("command line"), w2218, ":1200,n,8,1\"\n" ("command line")) -> (w2223:string)
                n1715 = Concatenate Strings(w2223, "CD\\\nCD WinDucom\nTIMEOUT 1\n bossac.exe -i -d --port=" ("command line"), w2218, " -U false -e -w -v -b DUE.bin -R\n" ("command line"), "\r") -> (w2225:string)
                "concatenated string 2" <- w2225
                n1716 = call <vilib>:"Write Characters To File.vi"("append to file? (new file:F)"=FALSE, "character string"=w2225, "file path (dialog if empty)"=path "C:/LAB-IQ-NXT/DUECOMPILE.bat" ("working directory")) -> ()  [unwired: 2 in, 1 out]
              }
              frame Enabled {
              }
            }
          }
          frame #2 {
            # "C:\\LAB-IQ-NXT\\DUECOMPILE.bat"
            n1717 = disable-structure shown="Disabled" {
              frame Disabled {
                w2230 = "cmd.exe  /c \"C:\\LAB-IQ-NXT\\DUECOMPILE.bat\"" ("string")
                n1718 = call <vilib>:"System Exec.vi"("expected output size  (4096)"=u32 65535, "run minimized? (F)"=FALSE, "wait until completion? (T)"=TRUE ("run minimized? (F)"), "working directory"=path "C:/LAB-IQ-NXT", "standard input"=w2230, "command line"=w2230) -> ("error out"=w2229:errorcluster, "standard output"=→"String 44":string)  [unwired: 2 in, 2 out]
                "error out 4" <- w2229
                n1719 = flat-sequence {
                  tunnel: w2229 -> [_]
                  frame #0 {
                  }
                }
              }
              frame Enabled {
              }
            }
            n1720 = local write "Prog Due"(FALSE ("Prog Due")) -> ()
          }
        }
      }
    }
    n1721 = Or(x=w1637, y=w1635) -> (x .or. y?=w1636:bool)
    n1722 = case shown="\"About\"" w1634 {
      tunnel: [T22."Acquire" ("Main Tab") T22."Compare Files" ("Main Tab") T22."About" ("Main Tab")] -> w1647
      frame "Acquire", Default {
      }
      frame "Compare Files" {
      }
      frame "About" {
      }
    }
    n1723 = Or(x=w1641, y="OPEN") -> (x .or. y?=w1642:bool)
    n1724 = case shown="True" w1642 {
      tunnel: w1641 -> [_ w1782]
      frame False {
      }
      frame True {
        n1725 = stacked-sequence {
          tunnel: w1782 -> [_ w1849 _ _]
          frame #0 {
            w1798 = "  " ("String 6")
            n1726 = local write "OPEN"(FALSE ("open")) -> ()
            n1727 = local read "string1 2"() -> (w1786:string)
            n1728 = local read "string1 3"() -> (w1785:string)
            n1729 = local read "string1 4"() -> (w1784:string)
            n1730 = property on="OPEN" class="Bool (strict)"("Visible"=FALSE) -> ()  [unwired: 2 in, 2 out]
            n1731 = local write "String 6"(w1798) -> ()
            n1732 = local write "String 7"(w1798) -> ()
            n1733 = local write "String 8"(w1798) -> ()
            n1734 = local write "String 12"(w1798) -> ()
            n1735 = local read "OK Button 16"() -> (w1783:bool)
            n1736 = String To Path(string=w1786) -> (path=w1794:path)
            n1737 = String To Path(string=w1785) -> (path=w1793:path)
            n1738 = String To Path(string=w1784) -> (path=w1792:path)
            n1739 = case shown="True" w1783 {
              tunnel: [w1799 w1800] -> w1787
              frame False {
                n1740 = local read "string1"() -> (w1799:string)
              }
              frame True {
                n1741 = local read "String Indicator 4"() -> (w1800:string)
              }
            }
            n1742 = Open/Create/Replace File "Open File"(file path (use dialog)=w1794) -> (refnum out=w1790:refnum<file>)  [unwired: 5 in, 2 out]
            n1743 = Open/Create/Replace File "Open File"(file path (use dialog)=w1793) -> (refnum out=w1789:refnum<file>)  [unwired: 5 in, 2 out]
            n1744 = Open/Create/Replace File "Open File"(file path (use dialog)=w1792) -> (refnum out=w1788:refnum<file>)  [unwired: 5 in, 2 out]
            n1745 = while {
              tunnel: w1790 -> [w1812]
              i -> [w1808]
              stop <- w1807 continue-if-true
              (unwired) TRUE ("line mode (F)")
              n1746 = Read from Text File "Read File"(file (use dialog)=w1812) -> (text=w1809:string)  [unwired: 3 in, 3 out]
              n1747 = local write "Numeric 11"(w1808) -> ()
              n1748 = String Length(string=w1809) -> (length=w1811:i32)
              n1749 = Greater?(x=w1811, y=1) -> (0:w1807:bool)
            }
            n1750 = while {
              tunnel: w1789 -> [w1818]
              i -> [w1814]
              stop <- w1813 continue-if-true
              (unwired) TRUE ("line mode (F)")
              n1751 = Read from Text File "Read File"(file (use dialog)=w1818) -> (text=w1815:string)  [unwired: 3 in, 3 out]
              n1752 = local write "Numeric 12"(w1814) -> ()
              n1753 = String Length(string=w1815) -> (length=w1817:i32)
              n1754 = Greater?(x=w1817, y=1) -> (0:w1813:bool)
            }
            n1755 = while {
              tunnel: w1788 -> [w1824]
              i -> [w1820]
              stop <- w1819 continue-if-true
              (unwired) TRUE ("line mode (F)")
              n1756 = Read from Text File "Read File"(file (use dialog)=w1824) -> (text=w1821:string)  [unwired: 3 in, 3 out]
              n1757 = local write "Numeric 13"(w1820) -> ()
              n1758 = String Length(string=w1821) -> (length=w1823:i32)
              n1759 = Greater?(x=w1823, y=1) -> (0:w1819:bool)
            }
            n1760 = String To Path(string=w1787) -> (path=w1795:path)
            n1761 = Open/Create/Replace File "Open File"(file path (use dialog)=w1795) -> (refnum out=w1791:refnum<file>)  [unwired: 5 in, 2 out]
            n1762 = while {
              tunnel: w1791 -> [w1806]
              i -> [w1802]
              stop <- w1801 continue-if-true
              (unwired) TRUE ("line mode (F)")
              n1763 = Read from Text File "Read File"(file (use dialog)=w1806) -> (text=w1803:string)  [unwired: 3 in, 3 out]
              n1764 = local write "Numeric 8"(w1802) -> ()
              n1765 = String Length(string=w1803) -> (length=w1805:i32)
              n1766 = Greater?(x=w1805, y=1) -> (0:w1801:bool)
            }
          }
          frame #1 {
            w1976 = FALSE ("ACTUAL   MERGE")
            # "Sample Temp"
            # "ECR"
            # "COF"
            # "Time\nCOF\nFF\nTemp"
            n1767 = case shown="True" w1849 {
              tunnel: [w1996 w1997] -> w1850
              frame False {
                n1768 = local read "string1"() -> (w1996:string)
              }
              frame True {
                n1769 = local read "String Indicator 4"() -> (w1997:string)
              }
            }
            n1770 = local read "string1 3"() -> (w1894:string)
            n1771 = String To Path(string=w1850) -> (path=w1981:path)
            n1772 = String To Path(string=w1894) -> (path=w1992:path)
            n1773 = local read "Numeric 12"() -> (w1978:i32)
            n1774 = local read "Numeric 8"() -> (w1980:i32)
            n1775 = local read "string1 2"() -> (w1895:string)
            n1776 = local read "string1 4"() -> (w1893:string)
            n1777 = Open/Create/Replace File "Open File"(file path (use dialog)=w1981) -> (refnum out=w1995:refnum<file>, error out=w1994:errorcluster)  [unwired: 5 in, 1 out]
            n1778 = Open/Create/Replace File "Open File"(file path (use dialog)=w1992) -> (refnum out=w1988:refnum<file>, error out=w1989:errorcluster)  [unwired: 5 in, 1 out]
            n1779 = for {
              N: w1980 -> [_]
              tunnel: w1995 -> [w2143]
              tunnel: w1994 -> [w2142]
              tunnel: [w2132] -> w1907 mode=indexing
              tunnel: [w2130] -> w1964 mode=indexing
              tunnel: [w2131] -> w1959 mode=indexing
              tunnel: w1976 -> [_]
              tunnel: [w2124] -> w1961 mode=indexing
              tunnel: [w2120] -> w1930 mode=indexing
              tunnel: [w2116] -> w1905 mode=indexing
              tunnel: [w2112] -> w1886 mode=indexing
              tunnel: [w2107] -> w1846 mode=indexing
              (unwired) TRUE ("line mode (F)")
              # "freq"
              # "Stroke"
              # "Time"
              # "CoF"
              # "Humidity"
              # "Temp"
              # "Air Temp"
              # "ECR"
              n1780 = Read from Text File "Read File"(file (use dialog)=w2143, error in=w2142) -> (text=w2108:string)  [unwired: 2 in, 3 out]
              n1781 = local write "String 6"(w2108) -> ()
              n1782 = String Subset(string=w2108, offset (0)=0, length (rest)=14 ("length (rest)")) -> (substring=w2136:string)
              n1783 = String Subset(string=w2108, offset (0)=35, length (rest)=9 ("length (rest)")) -> (substring=w2133:string)
              n1784 = String Subset(string=w2108, offset (0)=15, length (rest)=9 ("length (rest)")) -> (substring=w2139:string)
              n1785 = Fract/Exp String To Number(string=w2136) -> (number=w2132:dbl)  [unwired: 3 in, 1 out]
              n1786 = Fract/Exp String To Number(string=w2133) -> (number=w2131:dbl)  [unwired: 3 in, 1 out]
              n1787 = Fract/Exp String To Number(string=w2139) -> (number=w2130:dbl)  [unwired: 3 in, 1 out]
              n1788 = String Subset(string=w2108, offset (0)=85, length (rest)=9 ("length (rest)")) -> (substring=w2109:string)
              n1789 = String Subset(string=w2108, offset (0)=25, length (rest)=9 ("length (rest)")) -> (substring=w2115:string)
              n1790 = String Subset(string=w2108, offset (0)=55, length (rest)=9 ("length (rest)")) -> (substring=w2117:string)
              n1791 = String Subset(string=w2108, offset (0)=45, length (rest)=9 ("length (rest)")) -> (substring=w2123:string)
              n1792 = String Subset(string=w2108, offset (0)=65, length (rest)=9 ("length (rest)")) -> (substring=w2129:string)
              n1793 = Fract/Exp String To Number(string=w2115) -> (number=w2112:dbl)  [unwired: 3 in, 1 out]
              n1794 = Fract/Exp String To Number(string=w2109) -> (number=w2107:dbl)  [unwired: 3 in, 1 out]
              n1795 = Fract/Exp String To Number(string=w2117) -> (number=w2116:dbl)  [unwired: 3 in, 1 out]
              n1796 = Fract/Exp String To Number(string=w2123) -> (number=w2120:dbl)  [unwired: 3 in, 1 out]
              n1797 = Fract/Exp String To Number(string=w2129) -> (number=w2126:dbl)  [unwired: 3 in, 1 out]
              n1798 = Add(x=w2126, y=0.0) -> (x+y=w2124:dbl)
            }
            n1799 = for {
              N: w1978 -> [_]
              tunnel: w1989 -> [w2069]
              tunnel: w1988 -> [w2068]
              tunnel: [w2058] -> w1947 mode=indexing
              tunnel: [w2056] -> w1945 mode=indexing
              tunnel: [w2057] -> w1941 mode=indexing
              tunnel: w1976 -> [_]
              tunnel: [w2050] -> w1943 mode=indexing
              tunnel: [w2046] -> w1925 mode=indexing
              tunnel: [w2042] -> w1901 mode=indexing
              tunnel: [w2039] -> w1882 mode=indexing
              tunnel: [w2035] -> w1841 mode=indexing
              (unwired) 9 ("length (rest)")
              (unwired) 9 ("length (rest)")
              (unwired) TRUE ("line mode (F)")
              n1800 = Read from Text File "Read File"(file (use dialog)=w2068, error in=w2069) -> (text=w2036:string)  [unwired: 2 in, 3 out]
              n1801 = local write "String 8"(w2036) -> ()
              n1802 = String Subset(string=w2036, offset (0)=85) -> (substring=w2038:string)  [unwired: 1 in]
              n1803 = String Subset(string=w2036, offset (0)=35, length (rest)=9 ("length (rest)")) -> (substring=w2059:string)
